vi "TestExec.Operator Validation Check.vi"(11 "String":refnum<vi>) -> (1 "Description":string, 3 "OK":bool)   [LabVIEW 2018]
uses:
  <vilib>/KATE/Time/Time Utils.lvlib
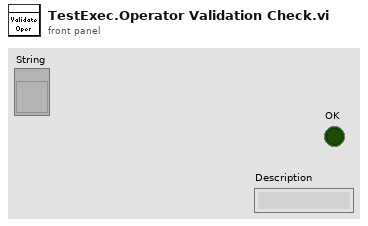
[diagram p1: front panel]
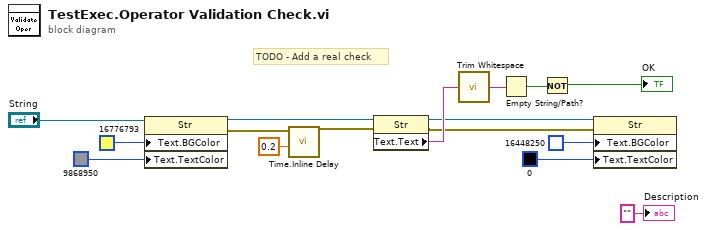
[diagram p0: block diagram]
diagram:
  # "TODO - Add a real check"
  n1 = property class="Str"(reference="String", "Text.BGColor"=u32 16776793, "Text.TextColor"=u32 9868950) -> (reference out=w8:refnum<vi>, error out=w15:errorcluster)  [unwired: 1 in]
  n2 = call <vilib>:"Time.Inline Delay.vi"("Wait(secs)"=0.2, "error in top"=w15) -> ("error out top"=w7:errorcluster)  [unwired: 8 in, 1 out]
  n3 = property class="Str"(reference=w8, error in=w7) -> (reference out=w4:refnum<vi>, error out=w3:errorcluster, "Text.Text"=w6:string)
  n4 = call <vilib>:"Trim Whitespace.vi"("string"=w6) -> ("trimmed string"=w5:string)  [unwired: 1 in]
  n5 = Empty String/Path?(string/path=w5) -> (empty?=w2:bool)
  n6 = Not(x=w2) -> (.not. x?=→"OK":bool)
  n7 = property class="Str"(reference=w4, error in=w3, "Text.BGColor"=u32 16448250, "Text.TextColor"=u32 0) -> ()  [unwired: 2 out]
  "Description" <- "" ("Description")
